vi "Convert Pointer To U8 Array.vi"(10 "Array Size":i32, 11 "Pointer":i32) -> (2 "U8 Array":u8[](array[numeric]), 3 "Pointer Out":u32)   [LabVIEW 2021]
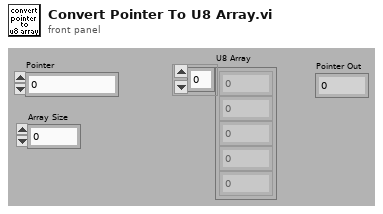
[diagram p1: front panel]
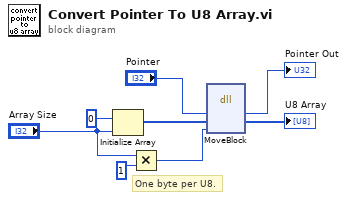
[diagram p0: block diagram]
diagram:
  # "One byte per U8."
  n1 = Initialize Array(u8 0 ("Element Data"), "Array Size") -> (w5:u8[])
  n2 = Multiply(x="Array Size", y=1) -> (x*y=w8:i32)
  n3 = dll-call lib="LabVIEW" fn="MoveBlock"("src"="Pointer", "dst"=w5, "size"=w8) -> ("src"=→"Pointer Out":u32, "dst"=→"U8 Array":u8[])  [unwired: 5 in, 2 out]
